vi "enable.vi"(8 "error in (no error)":errorcluster, 11 "Stimulator090724Scaffold in":refnum<class "Stimulator090724Scaffold.lvclass">) -> (0 "error out":errorcluster, 3 "Stimulator090724Scaffold out":refnum<class "Stimulator090724Scaffold.lvclass">)   [LabVIEW 2010, in "Stimulator090724Scaffold.lvclass"]
uses:
  Stimulator090724Scaffold.lvclass
  Stimulator090724Scaffold.lvclass/Stimulator090724Scaffold.ctl
  Clock/GenericClock/GenericClock/GenericClock.lvclass
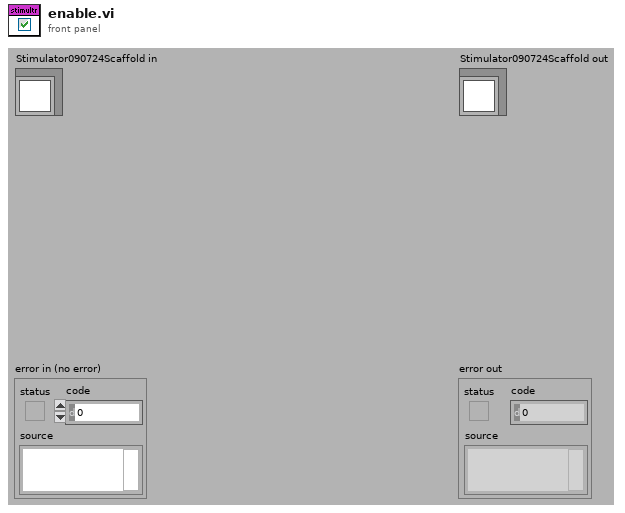
[diagram p1: front panel]
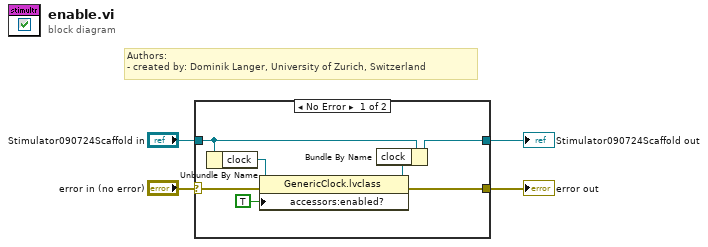
[diagram p0: block diagram]
diagram:
  # "Authors: \n- created by: Dominik Langer, University of Zurich, Switzerland"
  n1 = case shown="No Error" "error in (no error)" {
    selector: "error in (no error)" -> [w8 w12]
    tunnel: "Stimulator090724Scaffold in" -> [w11 w13]
    tunnel: [w7 w12] -> w2
    tunnel: [w10 w13] -> w1
    frame No Error {
      n2 = Unbundle By Name(w11) -> ("clock"=w9:refnum<class "GenericClock.lvclass">)
      n3 = property class="GenericClock.lvclass"(reference=w9, error in=w8, "accessors:enabled?"=TRUE ("enabled?")) -> (reference out=w6:refnum<class "GenericClock.lvclass">, error out=w7:errorcluster)
      n4 = Bundle By Name(cluster=w11, "clock"=w6) -> (w10:refnum<class "Stimulator090724Scaffold.lvclass">)
    }
    frame Error {
    }
  }
  "error out" <- w2
  "Stimulator090724Scaffold out" <- w1
